vi "Send Binary Data.vi"(8 "error in":errorcluster, 10 "Measurement Max and Min":dbl[](array[numeric]), 11 "VISA Refnum in":refnum<visa-resource-name>) -> (0 "error out":errorcluster, 3 "VISA Refnum out":refnum<visa-resource-name>)   [LabVIEW 2019]
doc: "Sends the \"Data\" message for use in the Binary examples."
uses:
  <vilib>/numeric/Random Number (Range) DBL.vi
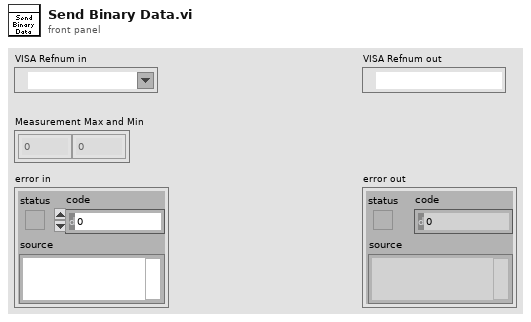
[diagram p1: front panel]
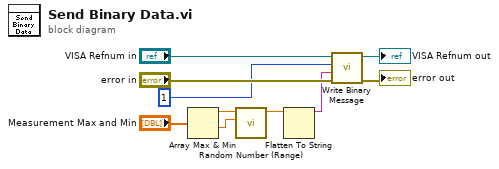
[diagram p0: block diagram]
diagram:
  n1 = Array Max & Min(array="Measurement Max and Min") -> (max value=w4:dbl, min value=w3:dbl)  [unwired: 2 out]
  n2 = call-poly <vilib>:"Random Number (Range).vi"("lower bound (0)"=w3, "upper bound (100)"=w4) -> ("number"=w2:dbl)  [unwired: 9 in]
  n3 = Flatten To String(anything=w2) -> (data string=w1:string)  [unwired: 3 in, 2 out]
  n4 = call "Write Binary Message.vi"("error in"="error in", "Flattened Data"=w1, "Message ID"=u8 1, "VISA resource in"="VISA Refnum in") -> ("error out"=→"error out":errorcluster, "VISA resource out"=→"VISA Refnum out":refnum<visa-resource-name>)  [unwired: 6 in]
